vi "Read Correct level .vi"(8 "error in (no error)":errorcluster, 11 "AM in":refnum<class "AM.lvclass">) -> (0 "error out":errorcluster, 2 "Correct level":bool, 3 "AM out":refnum<class "AM.lvclass">)   [LabVIEW 2020, in "AM.lvclass"]
uses:
  AM.lvclass
  AM.lvclass/AM.ctl
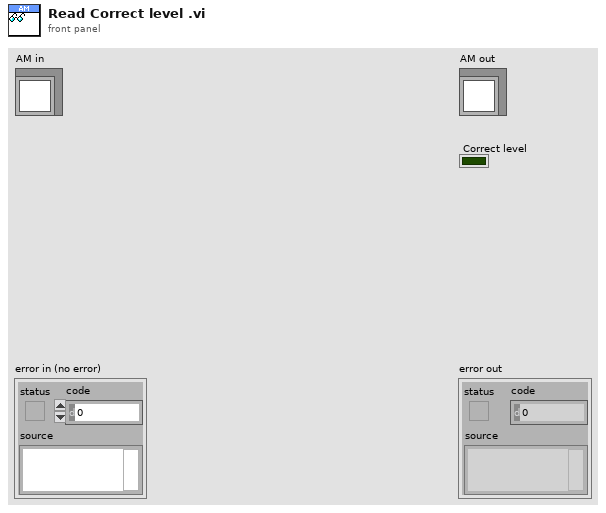
[diagram p1: front panel]
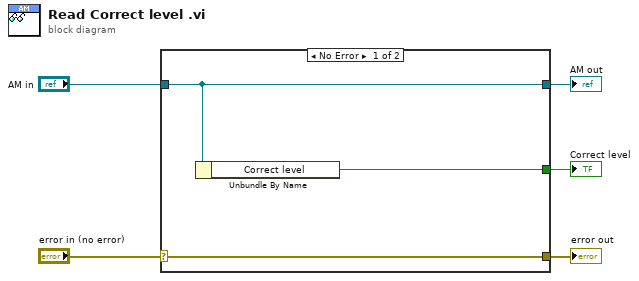
[diagram p0: block diagram]
diagram:
  n1 = case shown="No Error" "error in (no error)" {
    selector: "error in (no error)" -> [w8 w9]
    tunnel: [w8 w9] -> w4
    tunnel: [w7 w10] -> w2
    tunnel: "AM in" -> [w7 w10]
    tunnel: [w6 _] -> w1
    frame No Error {
      n2 = Unbundle By Name(w7) -> ("Correct level"=w6:bool)
    }
    frame Error {
    }
  }
  "error out" <- w4
  "AM out" <- w2
  "Correct level" <- w1
